vi "시스템로그.vi"(10 "이전 시스템 로그":string, 11 "진도 값":string) -> (3 "현재 시스템 로그":string)   [LabVIEW 2020]
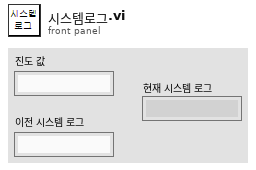
[diagram p1: front panel]
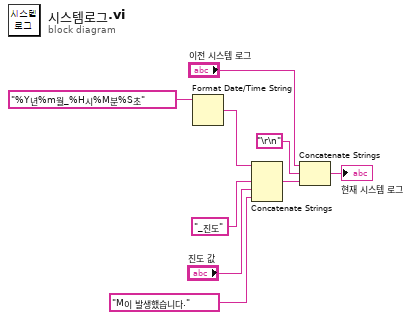
[diagram p0: block diagram]
diagram:
  n1 = Format Date/Time String(time format string (%c)="%Y년%m월_%H시%M분%S초" ("시간 포맷 문자열 (%c)")) -> (date/time string=w8:string)  [unwired: 2 in]
  n2 = Concatenate Strings(w8, "_진도", "진도 값", "M이 발생했습니다.") -> (w6:string)  [unwired: 1 in]
  n3 = Concatenate Strings("이전 시스템 로그", "\r\n", w6) -> (→"현재 시스템 로그":string)
